vi "Robo Command Stream Server.vi"(10 "StatusRefs":T1, 11 "Controller IP":string="192.168.1.199") -> ()   [LabVIEW 2015]
uses:
  Controls/RT Status Refs.ctl
  Robo Team Engine Command.ctl
  RT Controls/Generic instruction typedef.ctl
  RT Controls/RT Streamer Ack element.ctl
  Controls/LP Status typedef.ctl
  <vilib>/vision/Image Controls.llb/IMAQ Image.ctl
  <vilib>/dex/Flush And Wait Empty Condition.ctl
  Robo Team Globals.vi
  GUI/Host Globals.vi
  <resource>/objmgr/ni.dex.rc
panel:
  out "Close":bool
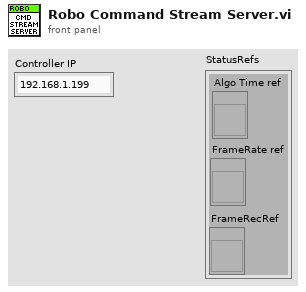
[diagram p1: front panel]
types:
  T1 = typedef "RT Status Refs.ctl" = cluster{"Algo Time ref":refnum<vi>, "FrameRate ref":refnum<vi>, "FrameRecRef":refnum<vi>}
  T2 = typedef "Generic instruction typedef.ctl" = cluster{"CMD":string, "Data":variant}
  T3 = typedef "Robo Team Engine Command.ctl" = cluster{"Command":string, "Data":variant, "Error":errorcluster, "Timeout":i32}
  T4 = typedef "LP Status typedef.ctl" = cluster{"FrameRate":dbl, "AlgoTime":dbl, "FrameRec":u16}
  T5 = typedef "RT Streamer Ack element.ctl" = cluster{"Data":variant, "CMD":string, "error":errorcluster}
  T6 = typedef "IMAQ Image.ctl" = refnum<image>
  T7 = typedef "Robo System State Refs.ctl" = cluster{"Engage Motor":refnum<vi>, "Auto Level":refnum<vi>, "IMU led":refnum<vi>, "Evaluate Enable":refnum<vi>, "Motor Led":refnum<vi>, "Error Descript":refnum<vi>, "Error Led":refnum<vi>, "Error":refnum<vi>}
  T8 = typedef "Flush And Wait Empty Condition.ctl" = u8
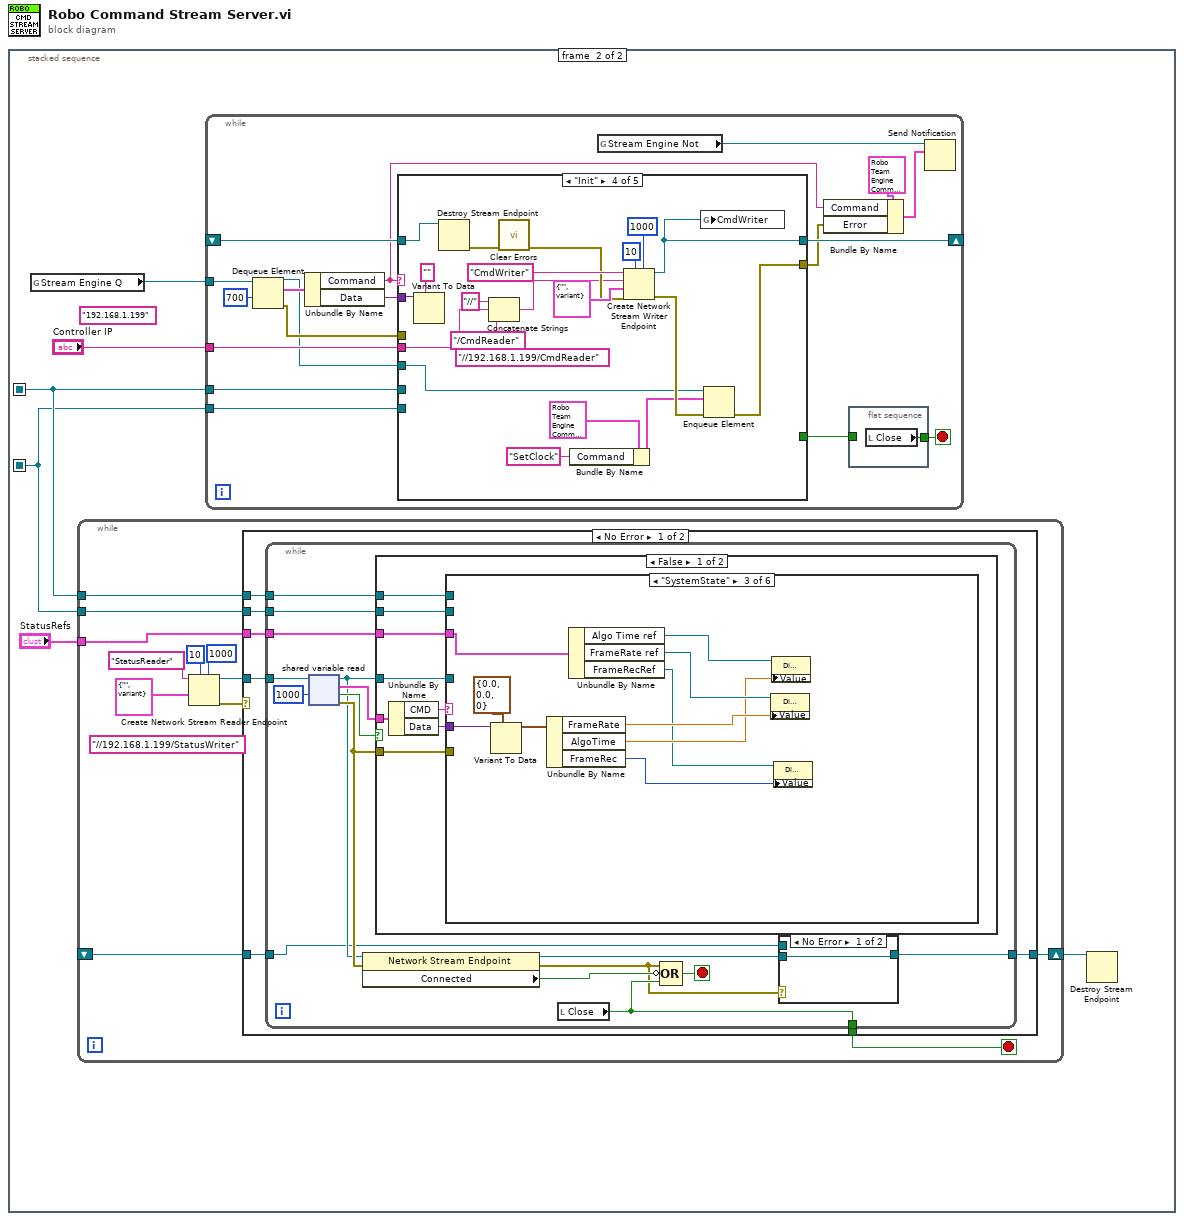
[diagram p0: block diagram]
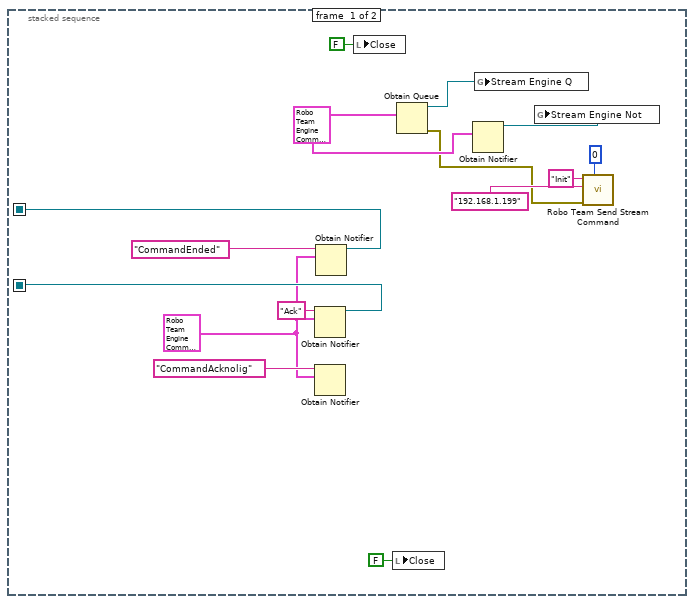
[diagram p2: hidden frame]
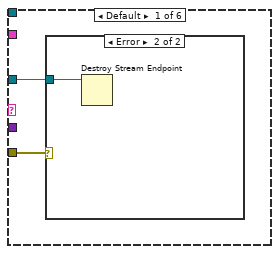
[diagram p4: hidden frame]
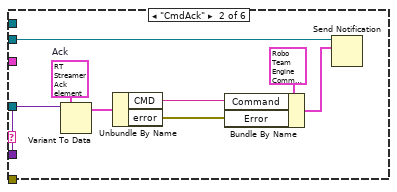
[diagram p6: hidden frame]
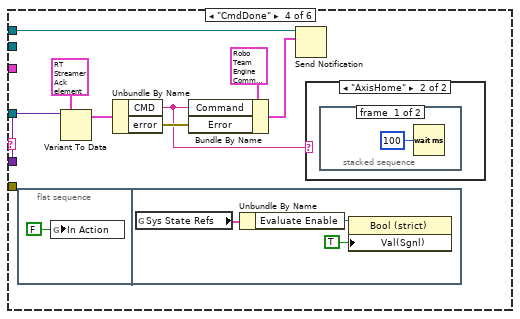
[diagram p7: hidden frame]
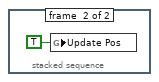
[diagram p9: hidden frame]
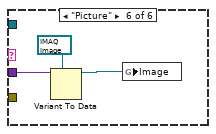
[diagram p11: hidden frame]
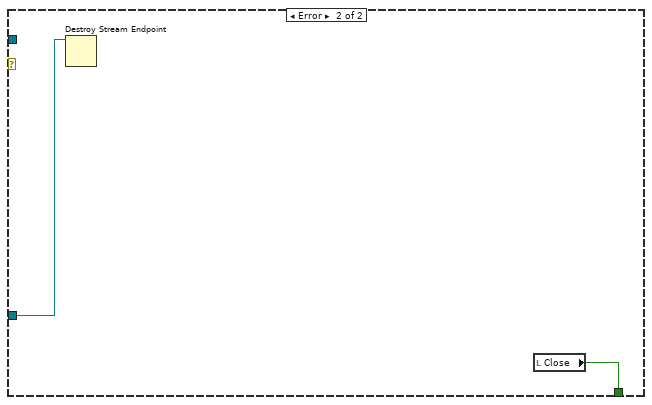
[diagram p13: hidden frame]
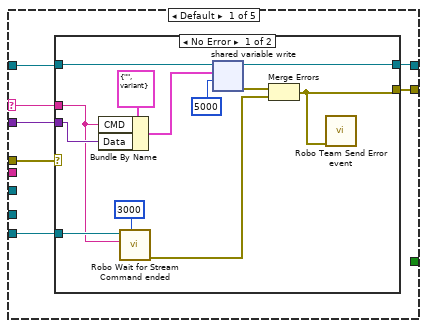
[diagram p14: hidden frame]
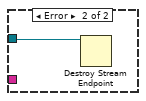
[diagram p15: hidden frame]
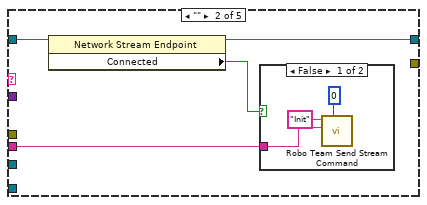
[diagram p16: hidden frame]
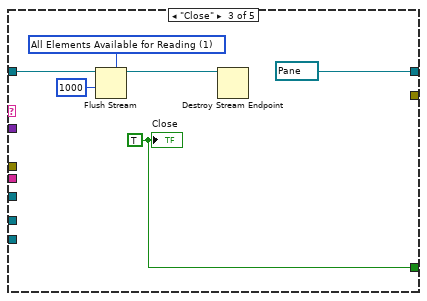
[diagram p18: hidden frame]
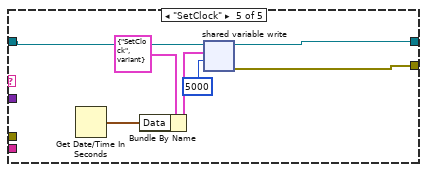
[diagram p19: hidden frame]
diagram:
  n1 = stacked-sequence {
    seq-local: [w13 _] -> [_ w20]
    seq-local: [w11 _] -> [_ w19]
    frame #0 {
      w7 = T3 {"Command"="", "Data"=variant, "Error"={"status"=FALSE, "code"=0, "source"=""}, "Timeout"=0} ("notification")
      w10 = T3 {"Command"="", "Data"=variant, "Error"={"status"=FALSE, "code"=0, "source"=""}, "Timeout"=0}
      n2 = Obtain Notifier(name (unnamed)="Ack", notification data type=w10) -> (notifier out=w11:refnum<notifier>)  [unwired: 2 in, 2 out]
      n3 = Obtain Notifier(name (unnamed)="CommandAcknolig", notification data type=w10) -> ()  [unwired: 2 in, 3 out]
      n4 = Obtain Notifier(name (unnamed)="CommandEnded", notification data type=w10) -> (notifier out=w13:refnum<notifier>)  [unwired: 2 in, 2 out]
      n5 = local write "Close"(FALSE ("Close")) -> ()
      n6 = local write "Close"(FALSE ("Close")) -> ()
      n7 = Obtain Queue(element data type=w7) -> (queue out=w6:refnum<queue>, error out=w1:errorcluster)  [unwired: 4 in, 1 out]
      n8 = Obtain Notifier(notification data type=w7) -> (notifier out=w5:refnum<notifier>)  [unwired: 3 in, 2 out]
      n9 = global write "Robo Team Globals.vi" "Stream Engine Q"(w6) -> ()
      n10 = global write "Robo Team Globals.vi" "Stream Engine Not"(w5) -> ()
      n11 = call "Robo Team Send Stream Command.vi"("timeout in ms (0)"=0 ("timeout in ms (5000)"), "error in (no error)"=w1, "Data in"="192.168.1.199" ("Command"), "Command"="Init") -> ()  [unwired: 6 in, 2 out]
    }
    frame #1 {
      (unwired) "192.168.1.199" ("Controller IP")
      n12 = global read "Robo Team Globals.vi" "Stream Engine Q"() -> (w21:refnum<queue>)
      n13 = while {
        tunnel: w20 -> [w28]
        tunnel: w19 -> [w26]
        shift-right: [w24] -> w17
        shift-left: _ -> [w23]
        tunnel: "StatusRefs" -> [w22]
        stop <- w27 stop-if-true
        (unwired) "//192.168.1.199/StatusWriter" ("Controller IP")
        n14 = Create Network Stream Reader Endpoint(5:1000 ("timeout in ms (-1)"), 7:10 ("reader buffer size"), 9:T2 {"CMD"="", "Data"=variant}, 11:"StatusReader" ("name (unnamed)")) -> (0:w25:errorcluster, 3:w31:refnum<k21>)  [unwired: 3 in]
        n15 = case shown="No Error" w25 {
          tunnel: w31 -> [w40 _]
          tunnel: w28 -> [w39 _]
          tunnel: [w38 w106] -> w27
          tunnel: w26 -> [w37 _]
          tunnel: [w36 _] -> w24
          tunnel: w23 -> [w35 w105]
          tunnel: w22 -> [w34 _]
          frame No Error {
            n16 = while {
              tunnel: w40 -> [w53]
              tunnel: w39 -> [w51]
              tunnel: [w50] -> w38
              tunnel: w37 -> [w49]
              tunnel: [w43] -> w36
              tunnel: w35 -> [w42]
              tunnel: w34 -> [w41]
              stop <- w54 stop-if-true
              n17 = shared-variable-read(w53, 1000 ("timeout ms (-1)")) -> (w46:refnum<k21>, w48:errorcluster, w55:bool, w56:T2)  [unwired: 1 in]
              n18 = property class="Network Stream Endpoint"(reference=w46, error in=w48) -> (reference out=w44:refnum<k21>, error out=w45:errorcluster, "Connected"=w47:bool)
              n19 = case shown="False" w55 {
                tunnel: w56 -> [w66 _]
                tunnel: w48 -> [w63 _]
                tunnel: w46 -> [w62 _]
                tunnel: w51 -> [w61 _]
                tunnel: w49 -> [w60 _]
                tunnel: w41 -> [w59 _]
                frame False {
                  n20 = Unbundle By Name(w66) -> ("CMD"=w65:string, "Data"=w64:variant)
                  n21 = case shown="\"SystemState\"" w65 {
                    tunnel: w64 -> [_ w77 w87 w95 _ w104]
                    tunnel: w63 -> [w68 _ _ _ _ _]
                    tunnel: w62 -> [w67 _ _ _ _ _]
                    tunnel: w61 -> [_ _ _ w90 _ _]
                    tunnel: w60 -> [_ w70 _ _ _ _]
                    tunnel: w59 -> [_ _ w85 _ _ _]
                    frame Default {
                      n22 = case shown="Error" w68 {
                        tunnel: w67 -> [_ w69]
                        frame No Error {
                        }
                        frame Error {
                          n23 = Destroy Stream Endpoint(11:w69) -> ()  [unwired: 1 in, 1 out]
                        }
                      }
                    }
                    frame "CmdAck" {
                      w76 = T5 {"Data"=variant, "CMD"="", "error"={"status"=FALSE, "code"=0, "source"=""}}  # Ack
                      n24 = Variant To Data(type=w76, Variant=w77) -> (data=w75:T5)  [unwired: 1 in, 1 out]
                      n25 = Unbundle By Name(w75) -> ("CMD"=w72:string, "error"=w71:errorcluster)
                      n26 = Bundle By Name(cluster=T3 {"Command"="", "Data"=variant, "Error"={"status"=FALSE, "code"=0, "source"=""}, "Timeout"=0} ("element"), "Command"=w72, "Error"=w71) -> (w73:T3)
                      n27 = Send Notification(notification=w73, notifier=w70) -> ()  [unwired: 1 in, 2 out]
                    }
                    frame "SystemState" {
                      n28 = Variant To Data(type=T4 {"FrameRate"=0.0, "AlgoTime"=0.0, "FrameRec"=0} ("LP Status"), Variant=w87) -> (data=w84:T4)  [unwired: 1 in, 1 out]
                      n29 = Unbundle By Name(w84) -> ("FrameRate"=w81:dbl, "AlgoTime"=w80:dbl, "FrameRec"=w78:u16)
                      n30 = Unbundle By Name(w85) -> ("Algo Time ref"=w83:refnum<vi>, "FrameRate ref"=w82:refnum<vi>, "FrameRecRef"=w79:refnum<vi>)
                      n31 = property class="DigNum (strict)"(reference=w82, "Value"=w81) -> ()  [unwired: 1 in, 2 out]
                      n32 = property class="DigNum (strict)"(reference=w83, "Value"=w80) -> ()  [unwired: 1 in, 2 out]
                      n33 = property class="DigNum (strict)"(reference=w79, "Value"=w78) -> ()  [unwired: 1 in, 2 out]
                    }
                    frame "CmdDone" {
                      n34 = flat-sequence {
                        frame #0 {
                          n35 = global write "Robo Team Globals.vi" "In Action"(FALSE ("In Action")) -> ()
                        }
                        frame #1 {
                          n36 = global read "Robo Team Globals.vi" "Sys State Refs"() -> (w99:T7)
                          n37 = Unbundle By Name(w99) -> ("Evaluate Enable"=w100:refnum<vi>)
                          n38 = property class="Bool (strict)"(reference=w100, "Val(Sgnl)"=TRUE ("Value (Signaling)")) -> ()  [unwired: 1 in, 2 out]
                        }
                      }
                      n39 = Variant To Data(type=T5 {"Data"=variant, "CMD"="", "error"={"status"=FALSE, "code"=0, "source"=""}} ("Ack"), Variant=w95) -> (data=w93:T5)  [unwired: 1 in, 1 out]
                      n40 = Unbundle By Name(w93) -> ("CMD"=w88:string, "error"=w91:errorcluster)
                      n41 = Bundle By Name(cluster=T3 {"Command"="", "Data"=variant, "Error"={"status"=FALSE, "code"=0, "source"=""}, "Timeout"=0} ("element"), "Command"=w88, "Error"=w91) -> (w89:T3)
                      n42 = Send Notification(notification=w89, notifier=w90) -> ()  [unwired: 1 in, 2 out]
                      n43 = case shown="\"AxisHome\"" w88 {
                        frame Default {
                        }
                        frame "AxisHome" {
                          n44 = stacked-sequence {
                            frame #0 {
                              n45 = Wait (ms)(milliseconds to wait=u32 100) -> ()  [unwired: 1 out]
                            }
                            frame #1 {
                              n46 = global write "Robo Team Globals.vi" "Update Pos"(TRUE ("Update Pos")) -> ()
                            }
                          }
                        }
                      }
                    }
                    frame "Status" {
                    }
                    frame "Picture" {
                      n47 = Variant To Data(type=T6 refnum ("Image"), Variant=w104) -> (data=w102:T6)  [unwired: 1 in, 1 out]
                      n48 = global write "Host Globals.vi" "Image"(w102) -> ()
                    }
                  }
                }
                frame True {
                }
              }
              n49 = local read "Close"() -> (w50:bool)
              n50 = Compound Arithmetic op=OR(w45, invert w47, w50) -> (w54:bool)
              n51 = case shown="No Error" w45 {
                tunnel: [w57 w58] -> w43
                tunnel: w44 -> [w57 _]
                tunnel: w42 -> [_ w58]
                frame No Error {
                }
                frame Error {
                }
              }
            }
          }
          frame Error {
            n52 = Destroy Stream Endpoint(11:w105) -> ()  [unwired: 1 in, 1 out]
            n53 = local read "Close"() -> (w106:bool)
          }
        }
      }
      n54 = while {
        tunnel: w21 -> [w124]
        shift-right: [w121] -> _
        shift-left: _ -> [w120]
        tunnel: w20 -> [w112]
        tunnel: w19 -> [w110]
        tunnel: "Controller IP" -> [w108]
        stop <- w113 stop-if-true
        n55 = Dequeue Element(queue=w124, timeout in ms (-1)=700) -> (queue out=w107:refnum<queue>, element=w123:T3, error out=w119:errorcluster)  [unwired: 1 in, 1 out]
        n56 = Unbundle By Name(w123) -> ("Command"=w115:string, "Data"=w122:variant)
        n57 = case shown="\"Init\"" w115 {
          selector: w115 -> [w129 _ _ _ _]
          tunnel: w122 -> [w128 _ _ w175 _]
          tunnel: [w130 w148 refnum<k21> refnum ("writer name") w167 w183] -> w121
          tunnel: w120 -> [w131 w149 w158 w171 w184]
          tunnel: w119 -> [w132 _ _ _ _]
          tunnel: [w126 _ _ w165 w179] -> w114
          tunnel: w112 -> [_ _ _ _ _]
          tunnel: [_ _ w156 _ _] -> w111
          tunnel: w110 -> [w127 _ _ _ _]
          tunnel: w108 -> [_ w146 _ w160 _]
          tunnel: w107 -> [_ _ _ w164 _]
          frame Default {
            n58 = case shown="No Error" w132 {
              tunnel: w131 -> [w143 w145]
              tunnel: [w142 _] -> w130
              tunnel: w129 -> [w136 _]
              tunnel: w128 -> [w139 _]
              tunnel: w127 -> [w137 _]
              tunnel: [w133 _] -> w126
              frame No Error {
                n59 = Bundle By Name(cluster=T2 {"CMD"="", "Data"=variant} ("data in"), "CMD"=w136, "Data"=w139) -> (w140:T2)
                n60 = call "Robo Wait for Stream Command ended.vi"("Timeout"=u32 3000, "Command"=w136, "Notifier in"=w137) -> ("error out"=w134:errorcluster)  [unwired: 8 in]
                n61 = shared-variable-write(w143, w140, 5000 ("timeout ms (-1)")) -> (w142:refnum<k21>, w135:errorcluster)  [unwired: 1 in, 1 out]
                n62 = Merge Errors(w135, w134) -> (w133:errorcluster)
                n63 = call "Robo Team Send Error event.vi"("error in (no error)"=w133) -> ()  [unwired: 11 in]
              }
              frame Error {
                n64 = Destroy Stream Endpoint(11:w145) -> ()  [unwired: 1 in, 1 out]
              }
            }
          }
          frame "" {
            n65 = property class="Network Stream Endpoint"(reference=w149) -> (reference out=w148:refnum<k21>, "Connected"=w147:bool)  [unwired: 1 in, 1 out]
            n66 = case shown="False" w147 {
              tunnel: w146 -> [w150 _]
              frame False {
                n67 = call "Robo Team Send Stream Command.vi"("timeout in ms (0)"=0 ("timeout in ms (5000)"), "Data in"=w150, "Command"="Init") -> ()  [unwired: 7 in, 2 out]
              }
              frame True {
              }
            }
          }
          frame "Close" {
            w154 = T8 1 items=["All Elements Read From Stream", "All Elements Available for Reading"] ("wait condition")
            w156 = TRUE ("Close")
            n68 = Flush Stream(9:1000 ("timeout in ms (-1)"), 10:w154, 11:w158) -> (3:w155:refnum<k21>)  [unwired: 1 in, 2 out]
            n69 = Destroy Stream Endpoint(11:w155) -> ()  [unwired: 1 in, 1 out]
            "Close" <- w156
          }
          frame "Init" {
            (unwired) "//192.168.1.199/CmdReader" ("Controller IP")
            n70 = Variant To Data(type="", Variant=w175) -> ()  [unwired: 1 in, 2 out]
            n71 = Destroy Stream Endpoint(11:w171) -> (0:w170:errorcluster)  [unwired: 1 in]
            n72 = Concatenate Strings("//" ("string"), w160, "/CmdReader" ("string")) -> (w159:string)
            n73 = call <vilib>:"Clear Errors.vi"("error in (no error)"=w170) -> ("error out"=w169:errorcluster)  [unwired: 5 in, 1 out]
            n74 = Bundle By Name(cluster=T3 {"Command"="", "Data"=variant, "Error"={"status"=FALSE, "code"=0, "source"=""}, "Timeout"=0} ("element"), "Command"="SetClock") -> (w162:T3)
            n75 = Create Network Stream Writer Endpoint(5:1000 ("timeout in ms (-1)"), 7:10 ("writer buffer size"), 8:w169, 9:T2 {"CMD"="", "Data"=variant}, 10:w159, 11:"CmdWriter" ("writer name")) -> (0:w166:errorcluster, 3:w167:refnum<k21>)  [unwired: 1 in]
            n76 = global write "Robo Team Globals.vi" "CmdWriter"(w167) -> ()
            n77 = Enqueue Element(queue=w164, element=w162, error in (no error)=w166) -> (error out=w165:errorcluster)  [unwired: 1 in, 2 out]
          }
          frame "SetClock" {
            n78 = Get Date/Time In Seconds() -> (seconds since 1Jan1904=w180:timestamp)
            n79 = Bundle By Name(cluster=T2 {"CMD"="SetClock", "Data"=variant} ("data in"), "Data"=w180) -> (w181:T2)
            n80 = shared-variable-write(w184, w181, 5000 ("timeout ms (-1)")) -> (w183:refnum<k21>, w179:errorcluster)  [unwired: 1 in, 1 out]
          }
        }
        n81 = global read "Robo Team Globals.vi" "Stream Engine Not"() -> (w118:refnum<notifier>)
        n82 = Bundle By Name(cluster=T3 {"Command"="", "Data"=variant, "Error"={"status"=FALSE, "code"=0, "source"=""}, "Timeout"=0} ("notification"), "Command"=w115, "Error"=w114) -> (w117:T3)
        n83 = flat-sequence {
          tunnel: [w125] -> w113
          tunnel: w111 -> [_]
          frame #0 {
            n84 = local read "Close"() -> (w125:bool)
          }
        }
        n85 = Send Notification(notification=w117, notifier=w118) -> ()  [unwired: 1 in, 2 out]
      }
      n86 = Destroy Stream Endpoint(11:w17) -> ()  [unwired: 1 in, 1 out]
    }
  }
